vi "CheckByteBoolean.vi"(1 "SingleByte":u8, 2 "StartIndex":u8) -> (7 "=10？":bool, 8 "=01？":bool)   [LabVIEW 2013]
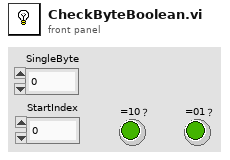
[diagram p1: front panel]
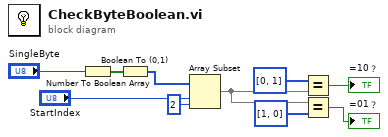
[diagram p0: block diagram]
diagram:
  n1 = Number To Boolean Array(number="SingleByte") -> (Boolean array=w10:bool[])
  n2 = Boolean To (0,1)(Boolean=w10) -> (0, 1=w9:i16[])
  n3 = Array Subset(array=w9, index="StartIndex", length=u8 2) -> (w6:i16[])
  n4 = Equal?(x=i16[] [0, 1], y=w6) -> (x = y?=→"=10？":bool)
  n5 = Equal?(x=w6, y=i16[] [1, 0] ("x")) -> (x = y?=→"=01？":bool)
